vi "que_wait_new_element.vi"(8 "error in (no error)":errorcluster, 11 "queue in":refnum<queue>) -> (0 "error out":errorcluster, 3 "queue out":refnum<queue>)   [LabVIEW 2013]
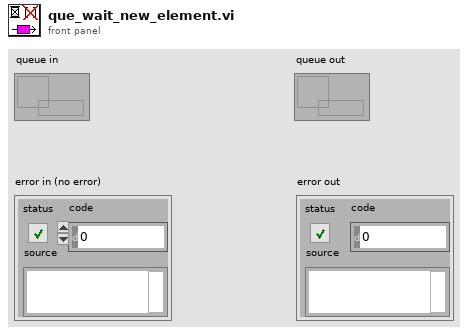
[diagram p1: front panel]
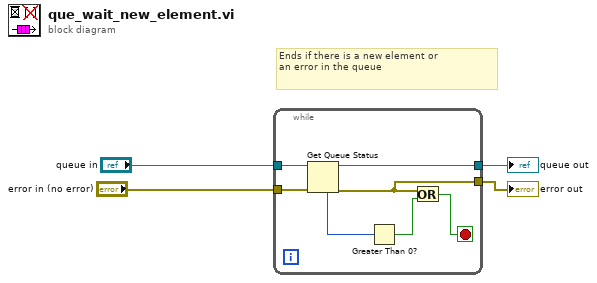
[diagram p0: block diagram]
diagram:
  # "Ends if there is a new element or\nan error in the queue"
  n1 = while {
    tunnel: "queue in" -> [w11]
    tunnel: "error in (no error)" -> [w9]
    tunnel: [w6] -> w4
    tunnel: [w5] -> w3
    stop <- w7 stop-if-true
    n2 = Get Queue Status(queue=w11, error in (no error)=w9) -> (queue out=w6:refnum<queue>, error out=w5:errorcluster, # elements in queue=w10:i32)  [unwired: 1 in, 5 out]
    n3 = Greater Than 0?(x=w10) -> (x > 0?=w8:bool)
    n4 = Or(x=w5, y=w8) -> (x .or. y?=w7:bool)
  }
  "queue out" <- w4
  "error out" <- w3
